vi "parseAutoShutDownErrorCodeShortStatus.vi"(8 "error in (no error)":errorcluster, 10 "shortStatus":string, 11 "DomeCommunicator in":refnum<class "ATDomeCommunicator.lvclass">) -> (0 "error out":errorcluster, 1 "sensorCode":T1, 2 "AutoShutdownON":bool, 3 "DomeCommunicator out":refnum<class "ATDomeCommunicator.lvclass">)   [LabVIEW 2016, in "ATDomeCommunicator.lvclass"]
uses:
  ATDomeCommunicator.lvclass
  ComTypedefs/sensorCode.ctl
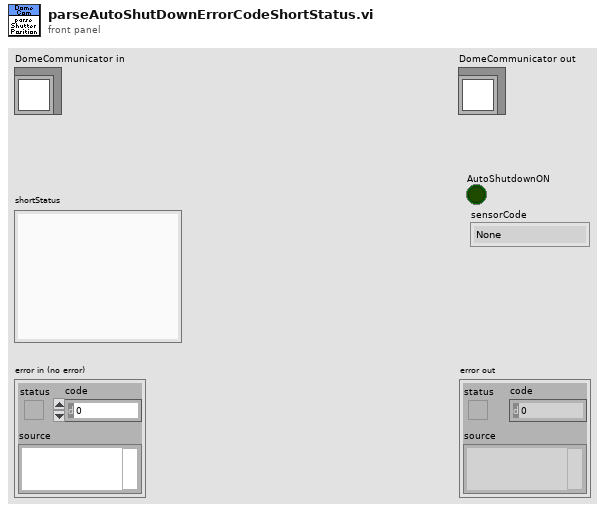
[diagram p1: front panel]
types:
  T1 = typedef "sensorCode.ctl" = enum16{"None", "RainSnowSensorTriggered", "CloudSensorTriggered", "BothSensorsTriggered"}
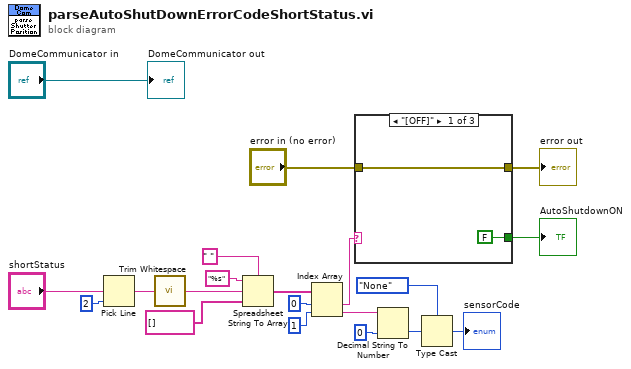
[diagram p0: block diagram]
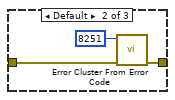
[diagram p2: hidden frame]
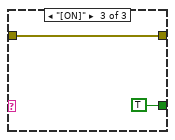
[diagram p3: hidden frame]
diagram:
  n1 = Pick Line(multi-line string="shortStatus", line index=2) -> (output string=w18:string)  [unwired: 1 in]
  n2 = call <vilib>:"Trim Whitespace.vi"("string"=w18) -> ("trimmed string"=w13:string)  [unwired: 1 in]
  n3 = Spreadsheet String To Array(delimiter (Tab)=" ", format string="%s", spreadsheet string=w13, array type (2D Dbl)=string[] []) -> (array=w9:string[])
  n4 = Index Array(array=w9, index #1=0 ("index"), index #2=1 ("index")) -> (element #1=w7:string, element #2=w4:string)
  n5 = case shown="\"[OFF]\"" w7 {
    tunnel: "error in (no error)" -> [w22 w24 w27]
    tunnel: [w22 w25 w27] -> w12
    tunnel: [FALSE ("Boolean") _ TRUE ("Boolean")] -> w1
    frame "[OFF]" {
    }
    frame Default {
      n6 = call <vilib>:"Error Cluster From Error Code.vi"("error in (no error)"=w24, "error code (0)"=8251) -> ("error out"=w25:errorcluster)  [unwired: 7 in]
    }
    frame "[ON]" {
    }
  }
  "error out" <- w12
  "AutoShutdownON" <- w1
  n7 = Decimal String To Number(string=w4, default (0L)=u16 0) -> (number=w3:u16)  [unwired: 1 in, 1 out]
  n8 = Type Cast(type=sensorCode."None" ("sensorCode"), x=w3) -> (*(type *) &x=→"sensorCode":T1)
  "DomeCommunicator out" <- "DomeCommunicator in"
